vi "SignalGenerate.vi"() -> ()   [LabVIEW 2014]
uses:
  <vilib>/express/express shared/transition.llb/Dynamic To Waveform Array.vi
  <vilib>/express/express arith-compare/Formula/Block/exnFormulaBlock how many pts in the wave.vi
  <vilib>/express/express shared/ex_Modify Signal Name.vi
  <vilib>/express/express shared/transition.llb/Waveform Array To Dynamic.vi
  <vilib>/express/express analysis/Spectral/Block/exnSpectralBlock spectral measurements peak poly.vi
  <vilib>/express/express analysis/Spectral/Block/exnSpectralBlock spectral measurements peak DDT.vi
  <vilib>/express/express arith-compare/Formula/XNode/ExpressFormulaBlockNode.xnode
  <vilib>/express/express analysis/Spectral/XNode/ExpressSpectralMeasurementsBlockNode.xnode
  <vilib>/ptbypt/NI_PtbyPt.lvlib
panel:
  in  "Trigger":bool
  out "Mean":dbl format="%0.2f"
  out "Peak to Peak":dbl
  out "Min Volts":dbl
  out "Max Volts":dbl
  out "Frequency":dbl
  out "Amplitude":dbl
  in  "WriteToFile":bool
  in  "Noise Type":string(combo)
  in  "Noise Control":dbl(knob)=1.0 caption="Amplitude" scale=0.0..5.0
  in  "Frequency Multiplier":dbl
  in  "Signal Type":string(combo)
  in  "DC Controller":dbl(knob) caption="Offset" scale=0.0..10.0
  in  "Amplitude":dbl(knob)=1.0 scale=0.0..100.0
  in  "Frequency":dbl(knob)=10.1 scale=0.0..200.0
  in  "?":enum32{"Oscillicope", "FFT "}(tab)
  in  "Show both cursors":bool
  in  "Volts/Div":i32(knob) scale=0.0..4.0
  in  "ms/Div":i32(knob) scale=0.0..4.0
  out "Oscilloscope Graph":dynamicdata(graph)
  out "FFT":dynamicdata(graph)
  in  "stop":bool
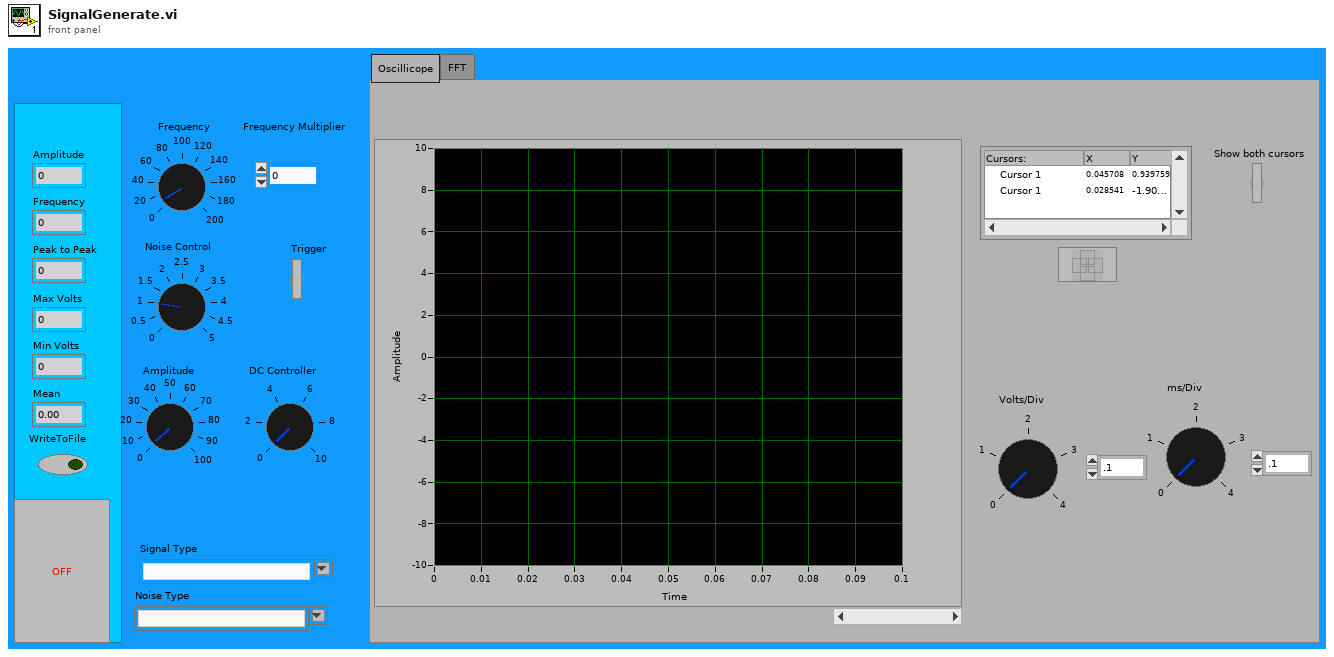
[diagram p1: front panel]
types:
  T1 = cluster{"averaging mode":u16, "weighting mode":u16, "number of averages":u32}
  T2 = cluster{"dB On (F)":bool, "unwrap phase (F)":bool, "convert to degree (F)":bool}
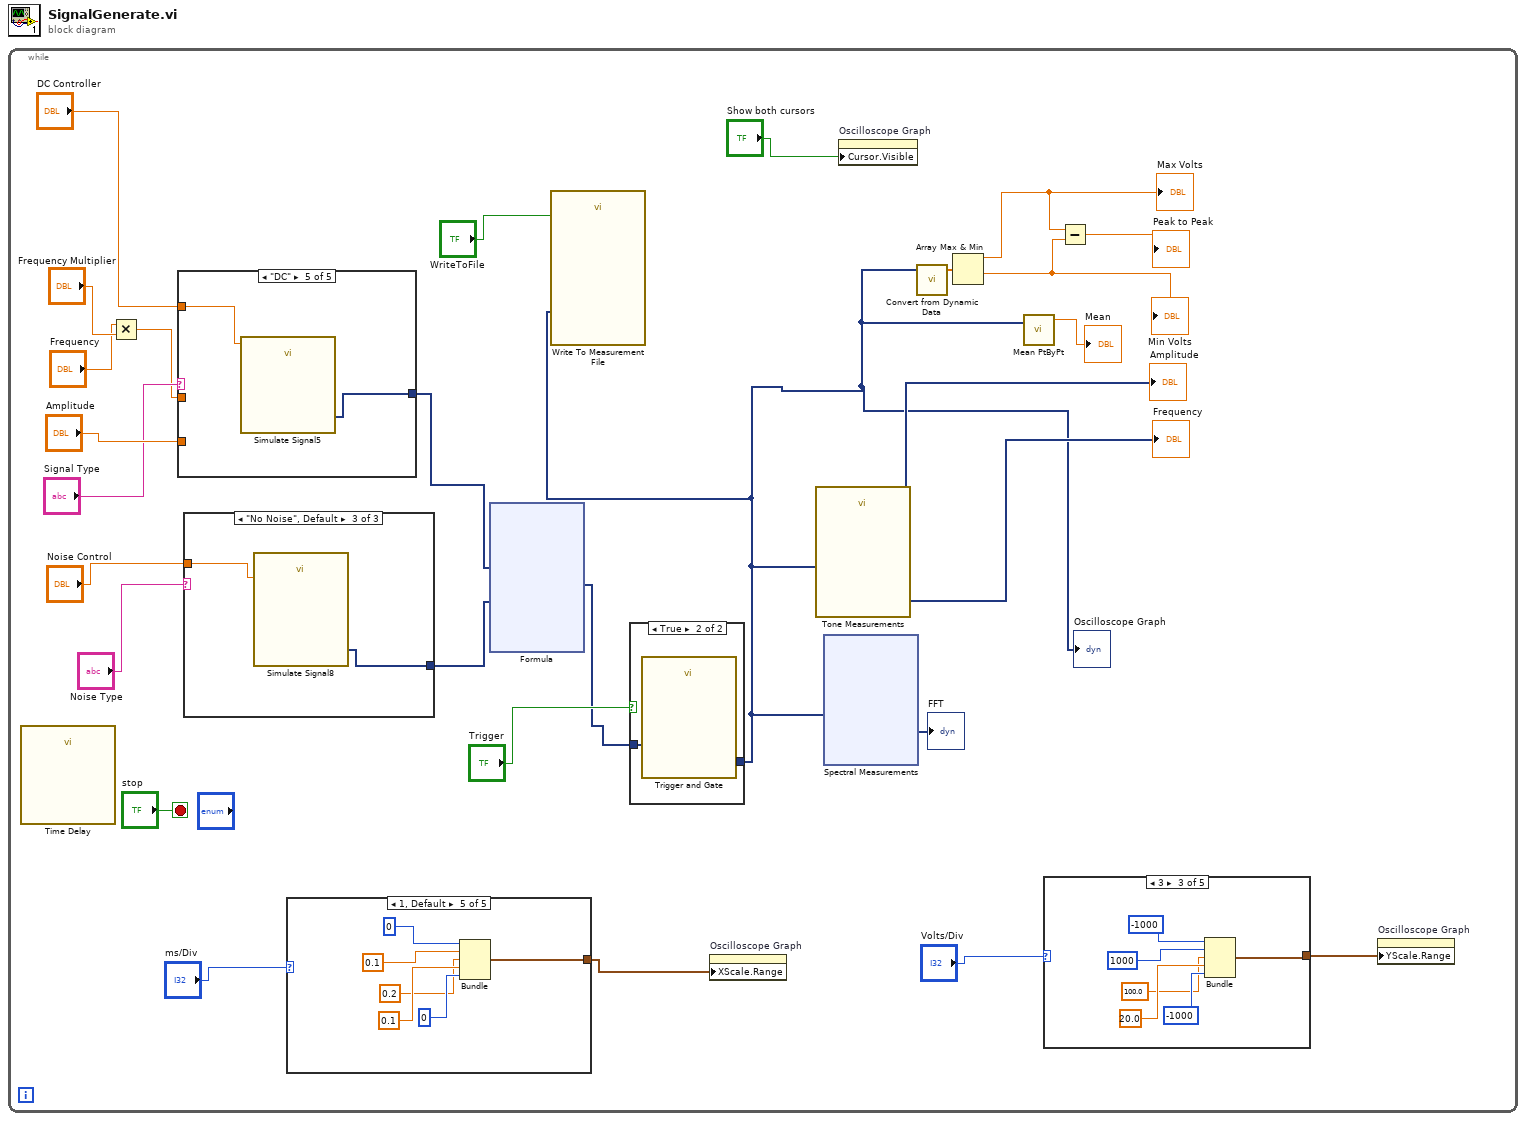
[diagram p0: block diagram]
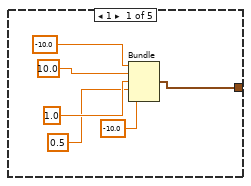
[diagram p2: hidden frame]
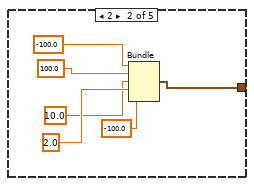
[diagram p3: hidden frame]
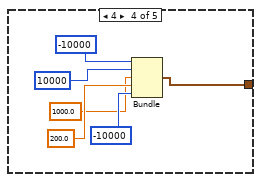
[diagram p4: hidden frame]
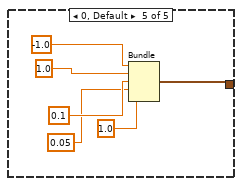
[diagram p5: hidden frame]
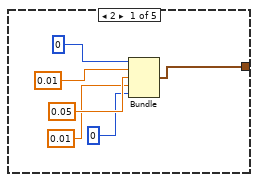
[diagram p6: hidden frame]
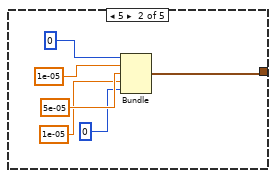
[diagram p7: hidden frame]
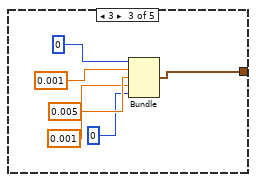
[diagram p8: hidden frame]
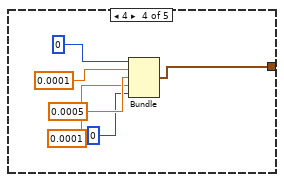
[diagram p9: hidden frame]
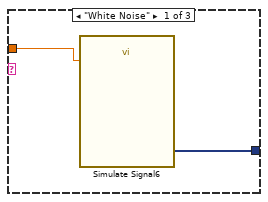
[diagram p11: hidden frame]
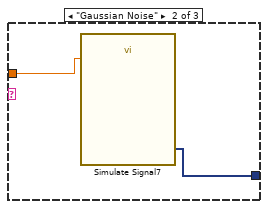
[diagram p12: hidden frame]
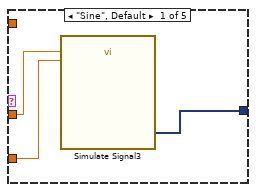
[diagram p13: hidden frame]
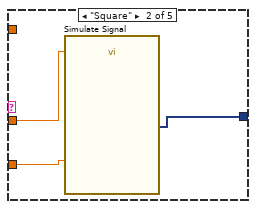
[diagram p14: hidden frame]
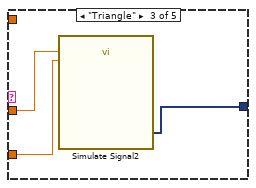
[diagram p15: hidden frame]
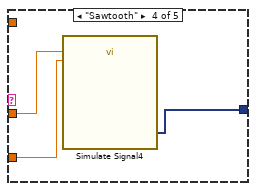
[diagram p16: hidden frame]
diagram:
  n1 = while {
    stop <- "stop" stop-if-true
    n2 = call "Time Delay"() -> ()  [unwired: 11 in, 1 out]
    n3 = Multiply(x="Frequency", y="Frequency Multiplier") -> (x*y=w23:dbl)
    n4 = case shown="\"DC\"" "Signal Type" {
      tunnel: [w249 w252 w255 w258 w260] -> w20
      tunnel: w23 -> [w247 w251 w253 w256 _]
      tunnel: "Amplitude" -> [w248 w250 w254 w257 _]
      tunnel: "DC Controller" -> [_ _ _ _ w259]
      frame "Sine", Default {
        n5 = call "Simulate Signal3"("Frequency"=w247, "Amplitude"=w248) -> ("Sine"=w249:dynamicdata)  [unwired: 12 in, 1 out]
      }
      frame "Square" {
        n6 = call "Simulate Signal"("Frequency"=w251, "Amplitude"=w250) -> ("Square"=w252:dynamicdata)  [unwired: 12 in, 1 out]
      }
      frame "Triangle" {
        n7 = call "Simulate Signal2"("Frequency"=w253, "Amplitude"=w254) -> ("Triangle"=w255:dynamicdata)  [unwired: 12 in, 1 out]
      }
      frame "Sawtooth" {
        n8 = call "Simulate Signal4"("Frequency"=w256, "Amplitude"=w257) -> ("Sawtooth"=w258:dynamicdata)  [unwired: 12 in, 1 out]
      }
      frame "DC" {
        n9 = call "Simulate Signal5"("Offset"=w259) -> ("DC"=w260:dynamicdata)  [unwired: 13 in, 1 out]
      }
    }
    n10 = case shown="\"No Noise\", Default" "Noise Type" {
      tunnel: "Noise Control" -> [w242 w244 w246]
      tunnel: [w241 w243 w245] -> w19
      frame "White Noise" {
        n11 = call "Simulate Signal6"("Amplitude"=w242) -> ("Sine with Uniform Noise"=w241:dynamicdata)  [unwired: 13 in, 1 out]
      }
      frame "Gaussian Noise" {
        n12 = call "Simulate Signal7"("Amplitude"=w244) -> ("Sine with Gaussian Noise"=w243:dynamicdata)  [unwired: 13 in, 1 out]
      }
      frame "No Noise", Default {
        n13 = call "Simulate Signal8"("Amplitude"=w246) -> ("Sine"=w245:dynamicdata)  [unwired: 13 in, 1 out]
      }
    }
    n14 = case shown="1, Default" "ms/Div" {
      tunnel: [w59 w65 w71 w77 w83] -> w4
      frame 2 {
        n15 = Bundle(0, 0.01, 0.05, 0.01, 0) -> (w59:cluster{i32, dbl, dbl, dbl, i32})  [unwired: 1 in]
      }
      frame 5 {
        n16 = Bundle(0, 1e-05, 5e-05, 1e-05, 0) -> (w65:cluster{i32, dbl, dbl, dbl, i32})  [unwired: 1 in]
      }
      frame 3 {
        n17 = Bundle(0, 0.001, 0.005, 0.001, 0) -> (w71:cluster{i32, dbl, dbl, dbl, i32})  [unwired: 1 in]
      }
      frame 4 {
        n18 = Bundle(0, 0.0001, 0.0005, 0.0001, 0) -> (w77:cluster{i32, dbl, dbl, dbl, i32})  [unwired: 1 in]
      }
      frame 1, Default {
        n19 = Bundle(0, 0.1, 0.2, 0.1, 0) -> (w83:cluster{i32, dbl, dbl, dbl, i32})  [unwired: 1 in]
      }
    }
    n20 = xnode "Formula"("No Noise"=w20, "Noise"=w19) -> ("Result"=w6:dynamicdata)  [unwired: 1 in, 1 out]
    n21 = case shown="True" "Trigger" {
      tunnel: w6 -> [w89 w91]
      tunnel: [w89 w90] -> w7
      frame False {
      }
      frame True {
        n22 = call "Trigger and Gate"("Signals"=w91) -> ("Triggered Signals"=w90:dynamicdata)  [unwired: 7 in, 3 out]
      }
    }
    "Oscilloscope Graph" <- w7
    n23 = call "Write To Measurement File"("Signals"=w7, "Enable"="WriteToFile") -> ()  [unwired: 15 in, 3 out]
    n24 = property on="Oscilloscope Graph" class="WFGraph (strict)"("XScale.Range"=w4) -> ()  [unwired: 2 in, 2 out]
    n25 = call "Tone Measurements"("Signals"=w7) -> ("Frequency"=→"Frequency":dynamicdata, "Amplitude"=→"Amplitude":dynamicdata)  [unwired: 8 in, 1 out]
    n26 = xnode "Spectral Measurements"("Signals"=w7) -> ("FFT - (Peak)"=→"FFT":dynamicdata)  [unwired: 1 in, 2 out]
    n27 = property on="Oscilloscope Graph" class="WFGraph (strict)"("Cursor.Visible"="Show both cursors") -> ()  [unwired: 2 in, 2 out]
    n28 = call "Convert from Dynamic Data"("Dynamic Data Type"=w7) -> ("Array"=w13:dbl[])  [unwired: 3 in]
    n29 = Array Max & Min(array=w13) -> (max value=w11:dbl, min value=w10:dbl)  [unwired: 2 out]
    "Max Volts" <- w11
    "Min Volts" <- w10
    n30 = call <vilib>:"Mean PtByPt.vi"("x"=w7) -> ("mean"=→"Mean":dbl)  [unwired: 3 in, 1 out]
    n31 = case shown="3" "Volts/Div" {
      tunnel: [w29 w38 w41 w47 w53] -> w3
      frame 1 {
        n32 = Bundle(-10.0, 10.0, 1.0, 0.5, -10.0) -> (w29:cluster{dbl, dbl, dbl, dbl, dbl})  [unwired: 1 in]
      }
      frame 2 {
        n33 = Bundle(-100.0, 100.0, 10.0, 2.0, -100.0) -> (w38:cluster{dbl, dbl, dbl, dbl, dbl})  [unwired: 1 in]
      }
      frame 3 {
        n34 = Bundle(-1000, 1000, 100.0, 20.0, -1000) -> (w41:cluster{i32, i32, dbl, dbl, i32})  [unwired: 1 in]
      }
      frame 4 {
        n35 = Bundle(-10000, 10000, 1000.0, 200.0, -10000) -> (w47:cluster{i32, i32, dbl, dbl, i32})  [unwired: 1 in]
      }
      frame 0, Default {
        n36 = Bundle(-1.0, 1.0, 0.1, 0.05, 1.0) -> (w53:cluster{dbl, dbl, dbl, dbl, dbl})  [unwired: 1 in]
      }
    }
    n37 = Subtract(x=w11, y=w10) -> (x-y=→"Peak to Peak":dbl)
    n38 = property on="Oscilloscope Graph" class="WFGraph (strict)"("YScale.Range"=w3) -> ()  [unwired: 2 in, 2 out]
  }
